vi "test_libssh2_sftp_mkdir_ex.vi"() -> ()   [LabVIEW 2013, in "libssh2_integration_tests.lvlib"]
uses:
  libssh2_integration_tests.lvlib
  <vilib>/addons/_JKI Toolkits/Caraya/classes/Test/Test.lvclass
  <vilib>/addons/_JKI Toolkits/Caraya/classes/Assert/Assert.lvclass
  libssh2/libssh2.lvlib
panel:
  out "error out":errorcluster
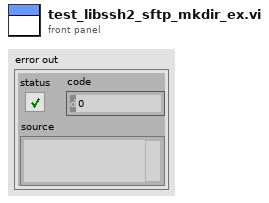
[diagram p1: front panel]
types:
  T1 = typedef "libssh2.lvlib/Session Refnum.ctl" = refnum<k1>
  T2 = typedef "libssh2.lvlib/SFTP Refnum.ctl" = refnum<k1>
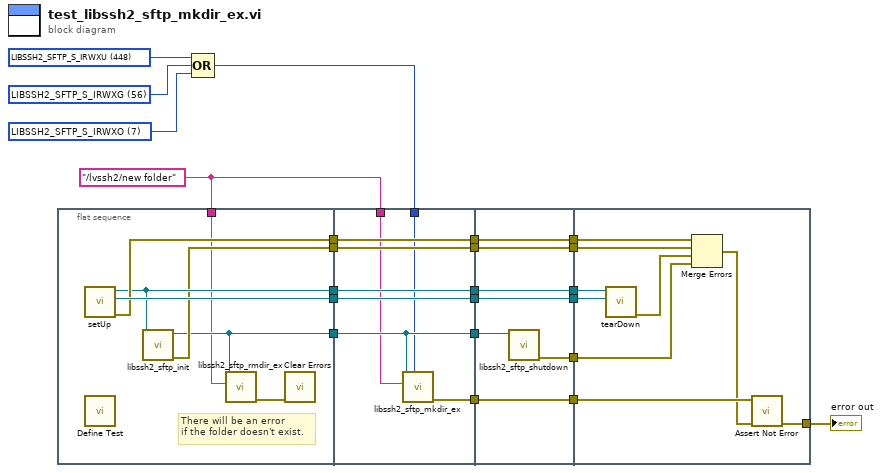
[diagram p0: block diagram]
diagram:
  w7 = "/lvssh2/new folder" ("filename")
  w15 = 7 items=["LIBSSH2_SFTP_S_IRWXU"=448, "LIBSSH2_SFTP_S_IRUSR"=256, "LIBSSH2_SFTP_S_IWUSR"=128, "LIBSSH2_SFTP_S_IXUSR"=64, "LIBSSH2_SFTP_S_IRWXG"=56, "LIBSSH2_SFTP_S_IRGRP"=32, "LIBSSH2_SFTP_S_IWGRP"=16, "LIBSSH2_SFTP_S_IXGRP"=8, "LIBSSH2_SFTP_S_IRWXO"=7, "LIBSSH2_SFTP_S_IROTH"=4, "LIBSSH2_SFTP_S_IWOTH"=2, "LIBSSH2_SFTP_S_IXOTH"=1] ("mode")
  w16 = 56 items=["LIBSSH2_SFTP_S_IRWXU"=448, "LIBSSH2_SFTP_S_IRUSR"=256, "LIBSSH2_SFTP_S_IWUSR"=128, "LIBSSH2_SFTP_S_IXUSR"=64, "LIBSSH2_SFTP_S_IRWXG"=56, "LIBSSH2_SFTP_S_IRGRP"=32, "LIBSSH2_SFTP_S_IWGRP"=16, "LIBSSH2_SFTP_S_IXGRP"=8, "LIBSSH2_SFTP_S_IRWXO"=7, "LIBSSH2_SFTP_S_IROTH"=4, "LIBSSH2_SFTP_S_IWOTH"=2, "LIBSSH2_SFTP_S_IXOTH"=1] ("mode")
  w17 = 448 items=["LIBSSH2_SFTP_S_IRWXU"=448, "LIBSSH2_SFTP_S_IRUSR"=256, "LIBSSH2_SFTP_S_IWUSR"=128, "LIBSSH2_SFTP_S_IXUSR"=64, "LIBSSH2_SFTP_S_IRWXG"=56, "LIBSSH2_SFTP_S_IRGRP"=32, "LIBSSH2_SFTP_S_IWGRP"=16, "LIBSSH2_SFTP_S_IXGRP"=8, "LIBSSH2_SFTP_S_IRWXO"=7, "LIBSSH2_SFTP_S_IROTH"=4, "LIBSSH2_SFTP_S_IWOTH"=2, "LIBSSH2_SFTP_S_IXOTH"=1] ("mode")
  n1 = flat-sequence {
    tunnel: [w28] -> w23
    tunnel: [w30] -> w22
    tunnel: [w29] -> w21
    tunnel: [w27] -> w19
    tunnel: [w26] -> w18
    tunnel: w7 -> [w25]
    tunnel: w23 -> [w38]
    tunnel: w22 -> [w37]
    tunnel: [w38] -> w6
    tunnel: [w37] -> w5
    tunnel: [w33] -> w4
    tunnel: [w34] -> w3
    tunnel: [w36] -> w2
    tunnel: w21 -> [w36]
    tunnel: w19 -> [w35]
    tunnel: [w35] -> w1
    tunnel: w18 -> [w33]
    tunnel: w14 -> [w32]
    tunnel: w7 -> [w31]
    tunnel: w6 -> [w45]
    tunnel: [w45] -> w13
    tunnel: w5 -> [w44]
    tunnel: [w44] -> w12
    tunnel: w4 -> [w40]
    tunnel: w3 -> [w43]
    tunnel: [w43] -> w11
    tunnel: w2 -> [w42]
    tunnel: [w42] -> w10
    tunnel: w1 -> [w41]
    tunnel: [w41] -> w9
    tunnel: [w39] -> w8
    tunnel: w13 -> [w54]
    tunnel: w12 -> [w53]
    tunnel: w11 -> [w52]
    tunnel: w10 -> [w51]
    tunnel: [w48] -> w20
    tunnel: w9 -> [w47]
    tunnel: w8 -> [w46]
    frame #0 {
      # "There will be an error\nif the folder doesn't exist."
      n2 = call "setUp.vi"() -> ("error out"=w29:errorcluster, "connection ID"=w30:refnum<k5>, "session"=w28:T1)  [unwired: 9 in]
      n3 = call <vilib>:"Define Test.vi"() -> ()  [unwired: 10 in, 2 out]
      n4 = call "libssh2_sftp_init.vi"("session"=w28) -> ("error out"=w27:errorcluster, "sftp"=w26:T2)  [unwired: 9 in]
      n5 = call "libssh2_sftp_rmdir_ex.vi"("path"=w25, "sftp"=w26) -> ("error out"=w24:errorcluster)  [unwired: 9 in]
      n6 = call <vilib>:"Clear Errors.vi"("error in (no error)"=w24) -> ()  [unwired: 6 in, 1 out]
    }
    frame #1 {
      n7 = call "libssh2_sftp_mkdir_ex.vi"("mode"=w32, "path"=w31, "sftp"=w33) -> ("error out"=w34:errorcluster)  [unwired: 8 in]
    }
    frame #2 {
      n8 = call "libssh2_sftp_shutdown.vi"("sftp"=w40) -> ("error out"=w39:errorcluster)  [unwired: 10 in]
    }
    frame #3 {
      n9 = call "tearDown.vi"("connection ID"=w53, "session"=w54) -> ("error out"=w50:errorcluster)  [unwired: 9 in]
      n10 = Merge Errors(w51, w47, w50, w46) -> (w49:errorcluster)
      n11 = call <vilib>:"Assert Not Error.vi"("error in (no error)"=w49, "Not Error?"=w52) -> ("error out"=w48:errorcluster)  [unwired: 8 in, 1 out]
    }
  }
  n12 = Compound Arithmetic op=OR(w17, w16, w15) -> (w14:i32)
  "error out" <- w20
